vi "AppendToGraph.vi"(6 "Enum":enum16{"XY", "XY2"}(ring), 8 "error in (no error)":errorcluster, 10 "wavenames":string[](array[string]), 11 "ITX Commands in":refnum<class "ITX Commands.lvclass">) -> (0 "error out":errorcluster, 3 "ITX Commands out":refnum<class "ITX Commands.lvclass">)   [LabVIEW 2016, in "ITX Commands.lvclass"]
uses:
  ITX Commands.lvclass
  ITX Commands.lvclass/ITX Commands.ctl
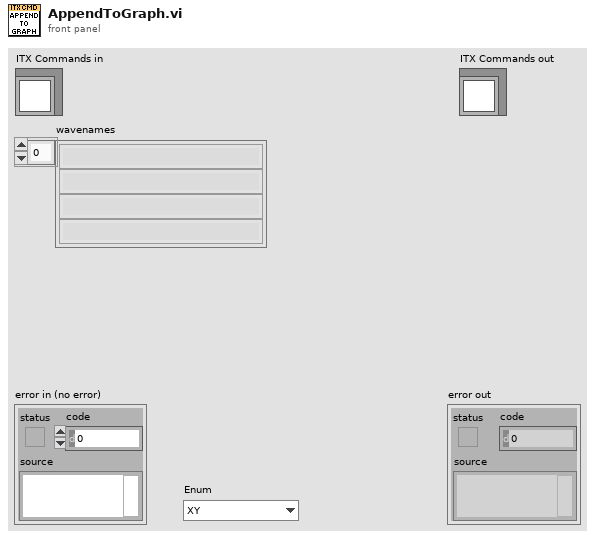
[diagram p1: front panel]
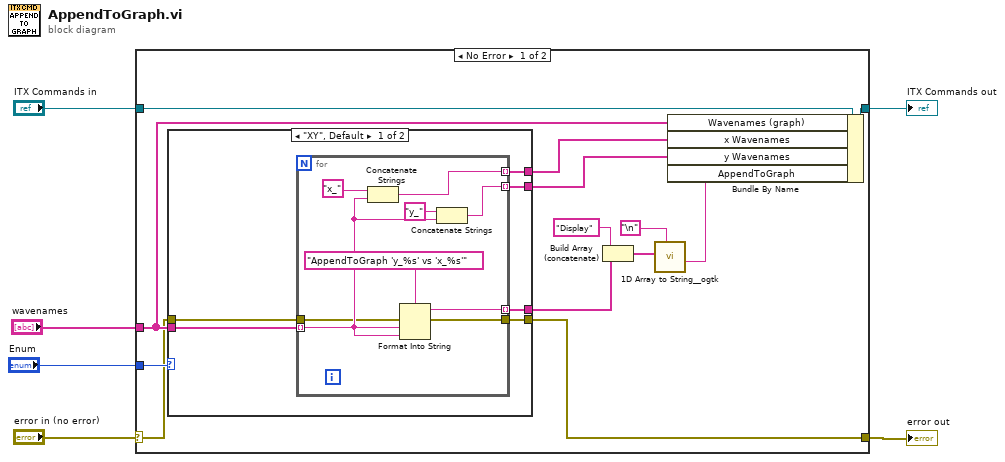
[diagram p0: block diagram]
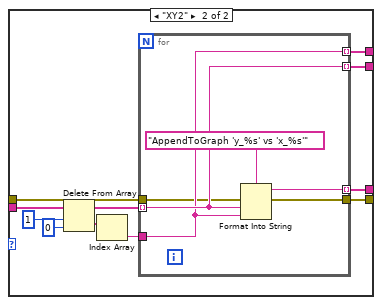
[diagram p2: hidden frame]
diagram:
  n1 = case shown="No Error" "error in (no error)" {
    selector: "error in (no error)" -> [w8 w53]
    tunnel: [w7 w53] -> w5
    tunnel: [w15 w52] -> w3
    tunnel: "ITX Commands in" -> [w16 w52]
    tunnel: "wavenames" -> [w12 _]
    tunnel: "Enum" -> [w13 _]
    frame No Error {
      n2 = case shown="\"XY\", Default" w13 {
        tunnel: [w25 w45] -> w19
        tunnel: w12 -> [w24 w42]
        tunnel: [w23 w44] -> w10
        tunnel: [w22 w43] -> w9
        tunnel: w8 -> [w20 w36]
        tunnel: [w21 w35] -> w7
        frame "XY", Default {
          n3 = for {
            tunnel: w24 -> [w33] mode=indexing
            tunnel: [w34] -> w25 mode=indexing
            tunnel: [w32] -> w23 mode=indexing
            tunnel: [w31] -> w22 mode=indexing
            tunnel: [w27] -> w21
            tunnel: w20 -> [w26]
            n4 = Concatenate Strings("x_", w33) -> (w32:string)
            n5 = Format Into String(format string="AppendToGraph 'y_%s' vs 'x_%s'", error in=w26, w33, w33) -> (resulting string=w34:string, error out=w27:errorcluster)  [unwired: 1 in]
            n6 = Concatenate Strings("y_", w33) -> (w31:string)
          }
        }
        frame "XY2" {
          n7 = Delete From Array(array=w42, length=1, index=0) -> (deleted portion=w41:string[], array with subset deleted=w38:string[])
          n8 = Index Array(array=w41) -> (element=w37:string)  [unwired: 1 in]
          n9 = for {
            tunnel: [w51] -> w45 mode=indexing
            tunnel: [w48] -> w44 mode=indexing
            tunnel: [w49] -> w43 mode=indexing
            tunnel: w37 -> [w48]
            tunnel: w38 -> [w49] mode=indexing
            tunnel: w36 -> [w47]
            tunnel: [w46] -> w35
            n10 = Format Into String(format string="AppendToGraph 'y_%s' vs 'x_%s'", error in=w47, w49, w48) -> (resulting string=w51:string, error out=w46:errorcluster)  [unwired: 1 in]
          }
        }
      }
      n11 = Build Array (concatenate)("Display", w19) -> (w17:string[])
      n12 = call <userlib>:"1D Array to String__ogtk.vi"("delimiter (Tab)"="\n", "Array of Strings"=w17) -> ("delimited string"=w11:string)  [unwired: 9 in]
      n13 = Bundle By Name(cluster=w16, "Wavenames (graph)"=w12, "x Wavenames"=w10, "y Wavenames"=w9, "AppendToGraph"=w11) -> (w15:refnum<class "ITX Commands.lvclass">)
    }
    frame Error {
    }
  }
  "error out" <- w5
  "ITX Commands out" <- w3
